vi "setLabelText.vi"(8 "error in (no error)":errorcluster, 10 "labelText":string, 11 "Wire in":refnum<class "Wire.lvclass">) -> (0 "error out":errorcluster, 3 "Wire out":refnum<class "Wire.lvclass">)   [LabVIEW 2023, in "TLC_Scripto.lvlib" / "Wire.lvclass"]
uses:
  Wire.lvclass
  TextDecoration/Write text.vi
  TextDecoration/Read textDecorationRef.vi
  TextDecoration/TextDecoration.lvclass
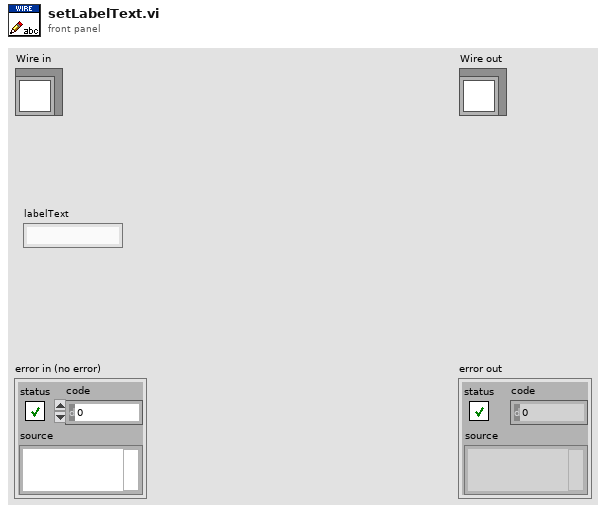
[diagram p1: front panel]
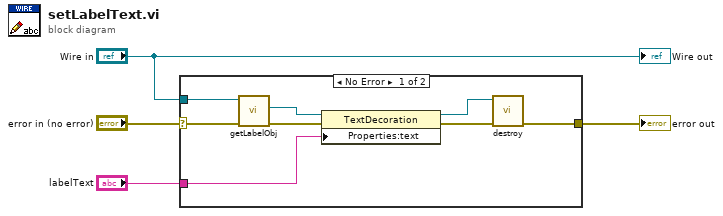
[diagram p0: block diagram]
diagram:
  n1 = case shown="No Error" "error in (no error)" {
    selector: "error in (no error)" -> [w11 w13]
    tunnel: "Wire in" -> [w12 _]
    tunnel: [w10 w13] -> w4
    tunnel: "labelText" -> [w5 _]
    frame No Error {
      n2 = call-dynamic "getLabelObj.vi"("error in (no error)"=w11, "Wire in"=w12) -> ("error out"=w9:errorcluster, "label"=w7:refnum<class "TextDecoration.lvclass">)  [unwired: 7 in, 1 out]
      n3 = property class="TextDecoration"(reference=w7, error in=w9, "Properties:text"=w5) -> (reference out=w6:refnum<class "TextDecoration.lvclass">, error out=w8:errorcluster)
      n4 = call-dynamic "destroy.vi"("Error In"=w8, "Generic In"=w6) -> ("Error Out"=w10:errorcluster)  [unwired: 9 in]
    }
    frame Error {
    }
  }
  "error out" <- w4
  "Wire out" <- "Wire in"
